vi "Write unit M.vi"(8 "Error In":errorcluster, 9 "Data In":bool, 10 "Position (U32)":u32, 11 "connection ID":refnum<k5>) -> (0 "Error Out":errorcluster, 3 "connection ID out":refnum<k5>)   [LabVIEW 2019, in "FX5U SLMP Binary.lvlib"]
uses:
  FX5U SLMP Binary.lvlib
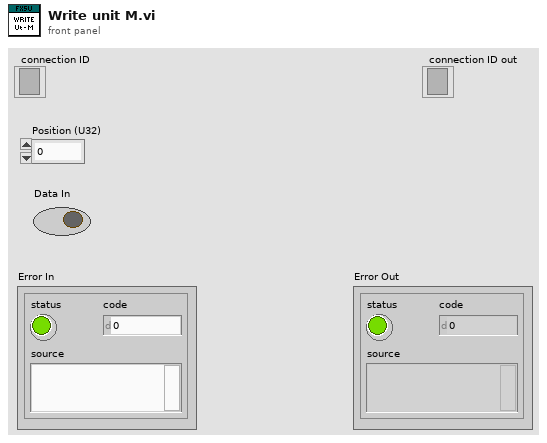
[diagram p1: front panel]
types:
  T1 = enum16{"big-endian, network order", "native, host order", "little-endian"}
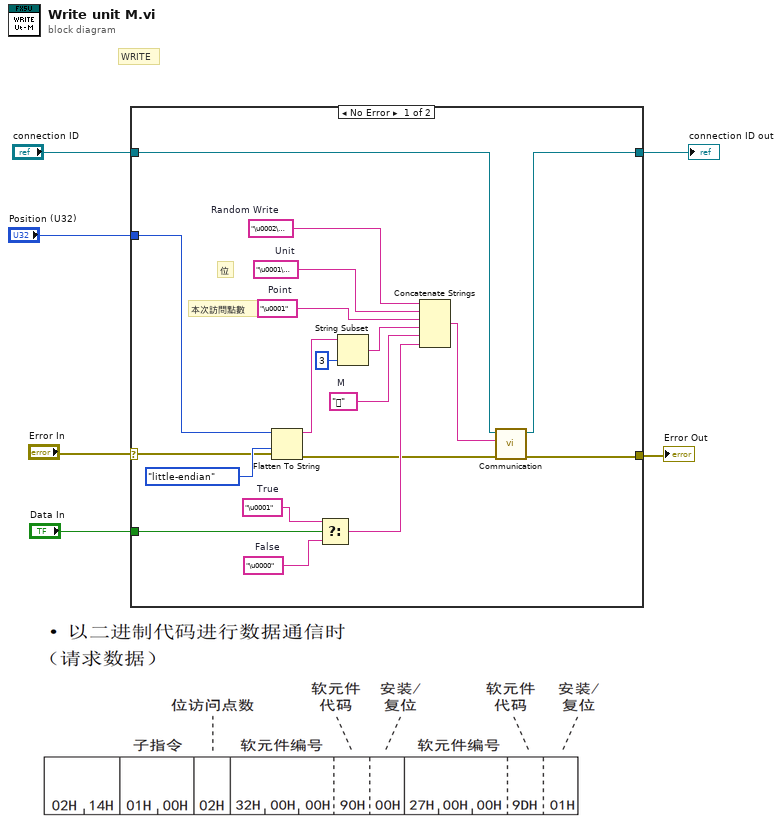
[diagram p0: block diagram]
diagram:
  # "WRITE"
  n1 = case shown="No Error" "Error In" {
    selector: "Error In" -> [w23 w27]
    tunnel: "Data In" -> [w22 _]
    tunnel: "Position (U32)" -> [w25 _]
    tunnel: [w10 w27] -> w3
    tunnel: "connection ID" -> [w9 w26]
    tunnel: [w8 w26] -> w1
    frame No Error {
      w13 = ""  # M
      w17 = "\u0001"  # Point
      w18 = "\u0001\u0000"  # Unit
      w19 = "\u0002\u0014"  # Random Write
      w20 = "\u0000"  # False
      w21 = "\u0001"  # True
      # "本次訪問點數"
      # "位"
      n2 = Flatten To String(anything=w25, byte order (0:big-endian, network order)=T1."little-endian", error in (no error)=w23) -> (data string=w16:string, error out=w11:errorcluster)  [unwired: 1 in, 1 out]
      n3 = Select(t=w21, s=w22, f=w20) -> (s? t:f=w12:string)
      n4 = String Subset(string=w16, length (rest)=3 ("length (rest)")) -> (substring=w14:string)  [unwired: 1 in]
      n5 = Concatenate Strings(w19, w18, w17, w14, w13, w12) -> (w7:string)
      n6 = call "Communication.vi"("Error In"=w11, "Command"=w7, "connection ID"=w9) -> ("Error Out"=w10:errorcluster, "connection ID out"=w8:refnum<k5>)  [unwired: 6 in, 1 out]
    }
    frame Error {
    }
  }
  "Error Out" <- w3
  "connection ID out" <- w1
